vi "Get Hwnd and Hide.vi"(0 "Doc Name":string, 5 "Shell Name":string, 11 "error in (no error)":errorcluster) -> (4 "Child hwnd":u32, 6 "Shell hwnd":u32, 15 "error out":errorcluster)   [LabVIEW 2016, in "Document.lvclass"]
uses:
  Document.lvclass
  user32.dll
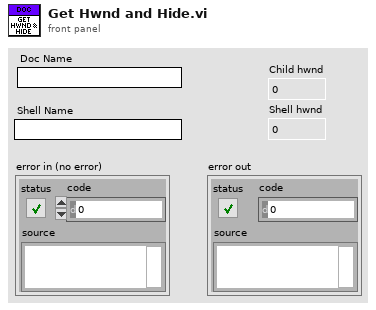
[diagram p1: front panel]
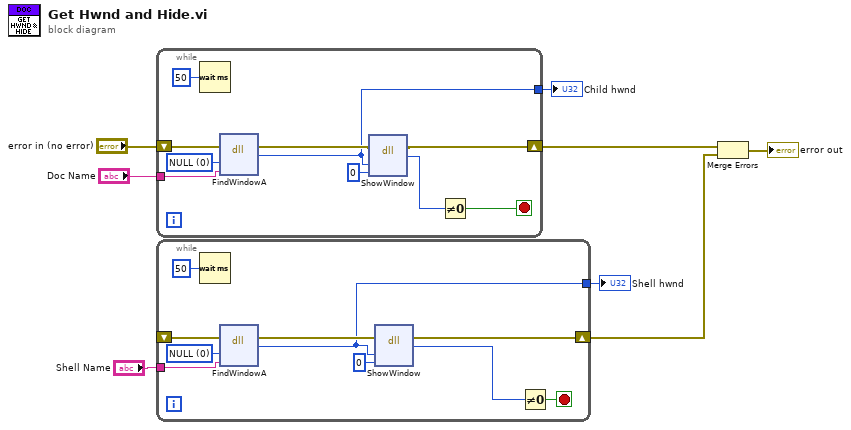
[diagram p0: block diagram]
diagram:
  n1 = while {
    tunnel: "Doc Name" -> [w16]
    shift-right: [w11] -> w5
    shift-left: "error in (no error)" -> [w17]
    tunnel: [w9] -> w2
    stop <- w14 stop-if-true
    w18 = 0 items=["NULL"]
    n2 = Wait (ms)(milliseconds to wait=u32 50) -> ()  [unwired: 1 out]
    n3 = dll-call lib="user32.dll" fn="FindWindowA"(error in=w17, "lpzsClassName"=w18, "lpzsWindowName"=w16) -> (error out=w12:errorcluster, "hwnd"=w9:u32)  [unwired: 4 in, 1 out]
    n4 = dll-call lib="user32.dll" fn="ShowWindow"(error in=w12, "hwnd"=w9, "nCmdShow"=u32 0) -> (error out=w11:errorcluster, "bool"=w10:u32)  [unwired: 4 in, 1 out]
    n5 = Not Equal To 0?(x=w10) -> (x != 0?=w14:bool)
  }
  "Child hwnd" <- w2
  n6 = while {
    tunnel: "Shell Name" -> [w25]
    shift-right: [w21] -> w4
    shift-left: _ -> [w26]
    tunnel: [w19] -> w1
    stop <- w23 stop-if-true
    w28 = 0 items=["NULL"]
    n7 = Wait (ms)(milliseconds to wait=u32 50) -> ()  [unwired: 1 out]
    n8 = dll-call lib="user32.dll" fn="FindWindowA"(error in=w26, "lpzsClassName"=w28, "lpzsWindowName"=w25) -> (error out=w27:errorcluster, "hwnd"=w19:u32)  [unwired: 4 in, 1 out]
    n9 = dll-call lib="user32.dll" fn="ShowWindow"(error in=w27, "hwnd"=w19, "nCmdShow"=u32 0) -> (error out=w21:errorcluster, "bool"=w20:u32)  [unwired: 4 in, 1 out]
    n10 = Not Equal To 0?(x=w20) -> (x != 0?=w23:bool)
  }
  "Shell hwnd" <- w1
  n11 = Merge Errors(w5, w4) -> (→"error out":errorcluster)
